vi "Terminate Std Out.vi"(4 "error in (no error)":errorcluster) -> (0 "error out":errorcluster)   [LabVIEW 2020, in "StdOut Operations.lvlib"]
uses:
  StdOut Operations.lvlib
  kernel32.dll
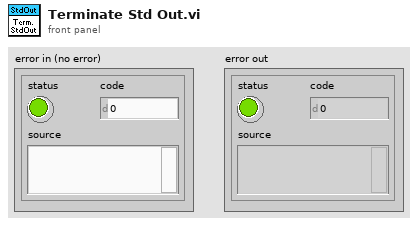
[diagram p1: front panel]
types:
  T1 = enum16{"Duplication Failed", "Duplication Succeeded"}
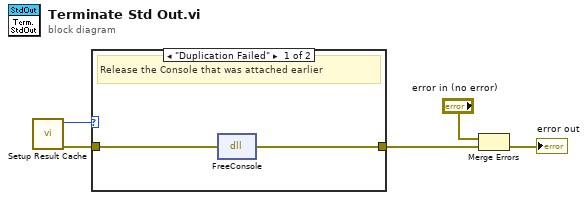
[diagram p0: block diagram]
diagram:
  n1 = call "Setup Result Cache.vi"() -> ("error out"=w2:errorcluster, "Result Out"=w1:T1)  [unwired: 7 in]
  n2 = case shown="\"Duplication Failed\"" w1 {
    tunnel: w2 -> [w7 w8]
    tunnel: [w6 w8] -> w5
    frame "Duplication Failed" {
      # "Release the Console that was attached earlier"
      n3 = dll-call lib="kernel32.dll" fn="FreeConsole"(error in=w7) -> (error out=w6:errorcluster)  [unwired: 2 in, 2 out]
    }
    frame "Duplication Succeeded" {
      # "Nothing to do, no attached console"
    }
  }
  n4 = Merge Errors("error in (no error)", w5) -> (→"error out":errorcluster)
